vi "GUI.vi"(9 "GUI Builder in":refnum<class "GUI Builder.lvclass">) -> ()   [LabVIEW 2021, in "App-Builder Library.lvlib" / "GUI Builder.lvclass"]
uses:
  GUI Builder.lvclass
  Builder/App descriptions.ctl
  Builder/Build Type.ctl
  GUI Builder.lvclass/GUI Builder.ctl
  Builder/Builder.lvclass
panel:
  in  "Application found":T1[](array[typedef])
  out "update":bool
  in  "Build button":bool
  # "Build Name"
  # "Type"
  # "Current Version"
  # "Next Version"
  # "Build?"
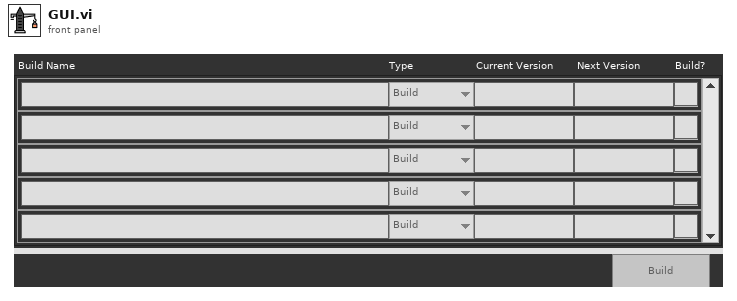
[diagram p1: front panel]
types:
  T1 = typedef "App-Builder Library.lvlib/Builder.lvclass/App descriptions.ctl" = cluster{"App Name":string, "Build Type":T2, "Current Version":string, "Next Version":string, "Check":bool}
  T2 = typedef "App-Builder Library.lvlib/Builder.lvclass/Build Type.ctl" = enum16{"Major", "Minor", "Fix", "Build"}
  T3 = enum8{"Enabled", "Disabled", "Disabled and Grayed Out"}
  T4 = typedef "NI_App_Builder_API.lvlib/Build Specification Version.ctl" = cluster{"Major":u16, "Minor":u16, "Fix":u16, "Build":u16}
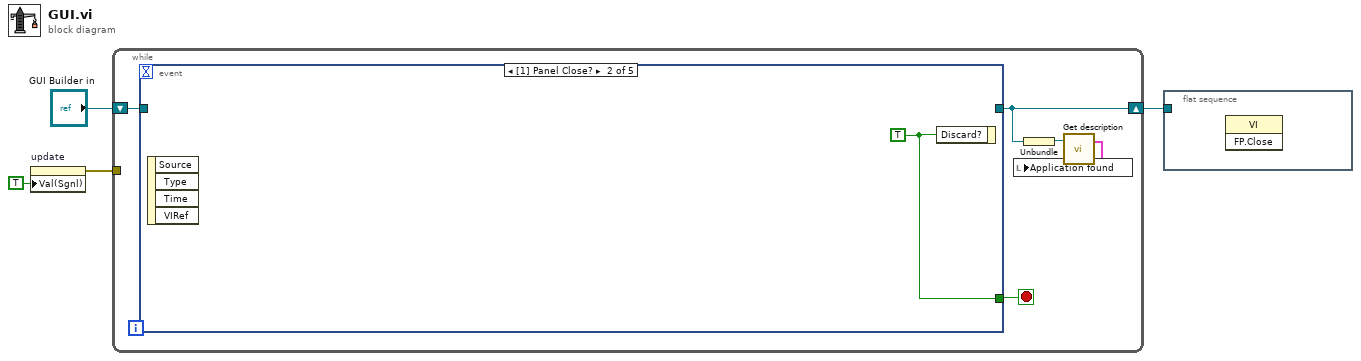
[diagram p0: block diagram]
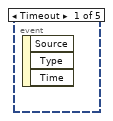
[diagram p2: hidden frame]
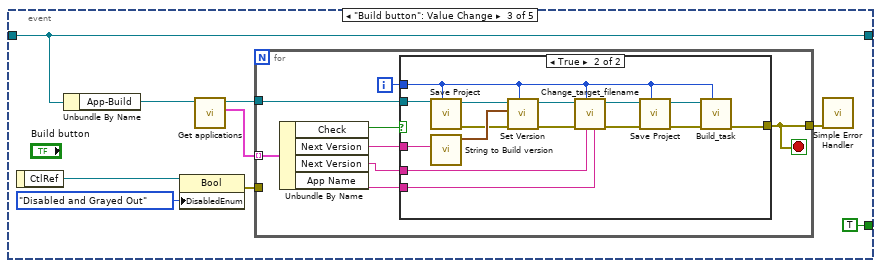
[diagram p3: hidden frame]
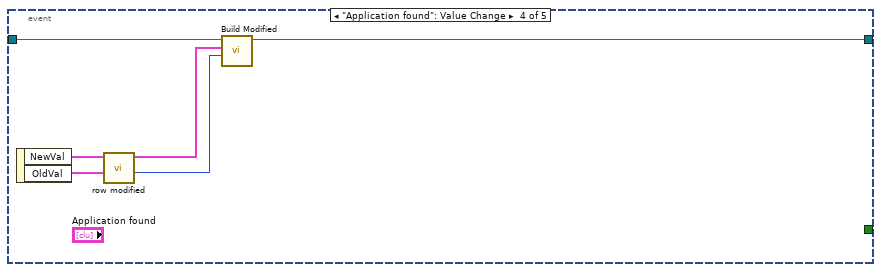
[diagram p5: hidden frame]
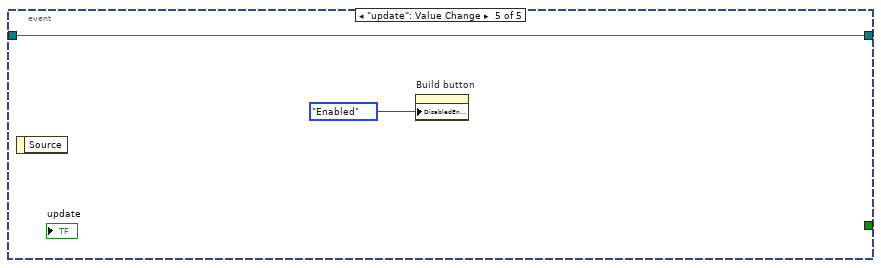
[diagram p6: hidden frame]
diagram:
  n1 = property on="update" class="Bool (strict)"("Val(Sgnl)"=TRUE ("Value (Signaling)")) -> (error out=w2:errorcluster)  [unwired: 2 in, 1 out]
  n2 = while {
    shift-right: [w6] -> w1
    shift-left: "GUI Builder in" -> [w8]
    tunnel: w2 -> [_]
    stop <- w9 stop-if-true
    n3 = event shown="[1] Panel Close?" {
      selector: _ -> [_ _ _ _ _]
      dyn-events: _ -> [_ _ _ _ _]
      timeout: _ -> [_ _ _ _ _]
      tunnel: [_ w10 TRUE ("Discard?") _ _] -> w9
      tunnel: w8 -> [_ _ w19 w46 w50]
      tunnel: [_ _ w19 w44 w50] -> w6
      event Timeout {
        n4 = event-data() -> ()  [unwired: 1 in, 3 out]
      }
      event Panel Close? {
        w10 = TRUE ("Discard?")
        n5 = event-data() -> ()  [unwired: 1 in, 4 out]
        n6 = event-data("Discard?"=w10) -> ()  [unwired: 1 in, 1 out]
      }
      event "Build button": Value Change {
        n7 = event-data() -> ("CtlRef"=w15:refnum<vi>)  [unwired: 1 in]
        n8 = Unbundle By Name(w19) -> ("App-Build"=w18:refnum<class "Builder.lvclass">)
        n9 = property class="Bool"(reference=w15, "DisabledEnum"=T3."Disabled and Grayed Out" ("Disabled")) -> (error out=w13:errorcluster)  [unwired: 1 in, 1 out]
        n10 = call "Get applications.vi"("Builder in"=w18) -> ("Applications"=w16:T1[], "Builder out"=w17:refnum<class "Builder.lvclass">)  [unwired: 9 in]
        n11 = for {
          tunnel: [w22] -> w11
          tunnel: w17 -> [w27]
          tunnel: w16 -> [w26] mode=indexing
          tunnel: w13 -> [_]
          i -> [w24]
          stop <- w22 stop-if-true
          n12 = Unbundle By Name(w26) -> ("Check"=w25:bool, "Next Version"=w23:string, "Next Version"=w20:string, "App Name"=w21:string)
          n13 = case shown="True" w25 {
            tunnel: [_ w32] -> w22
            tunnel: w27 -> [_ w38]
            tunnel: w24 -> [_ w30]
            tunnel: w23 -> [_ w40]
            tunnel: w21 -> [_ w29]
            tunnel: w20 -> [_ w28]
            frame False {
            }
            frame True {
              n14 = call "Save Project.vi"("index"=w30, "Builder in"=w38) -> ("error out"=w31:errorcluster, "Builder out"=w37:refnum<class "Builder.lvclass">)  [unwired: 8 in]
              n15 = call "String to Build version.vi"("Build Version (String)"=w40) -> ("Build Version"=w39:T4)  [unwired: 10 in]
              n16 = call "Set Version.vi"("Index"=w30, "error in"=w31, "Build Version"=w39, "Builder in"=w37) -> ("error out"=w41:errorcluster, "Builder out"=w42:refnum<class "Builder.lvclass">)  [unwired: 6 in]
              n17 = call "Change_target_filename.vi"("App Name"=w29, "New Version"=w28, "index"=w30, "error in (no error)"=w41, "Builder in"=w42) -> ("error out"=w36:errorcluster, "Builder out"=w35:refnum<class "Builder.lvclass">)  [unwired: 5 in]
              n18 = call "Save Project.vi"("index"=w30, "error in"=w36, "Builder in"=w35) -> ("error out"=w33:errorcluster, "Builder out"=w34:refnum<class "Builder.lvclass">)  [unwired: 7 in]
              n19 = call "Build_task.vi"("index"=w30, "error in"=w33, "Builder in"=w34) -> ("error out"=w32:errorcluster)  [unwired: 6 in, 2 out]
            }
          }
        }
        n20 = call <vilib>:"Simple Error Handler.vi"("error in (no error)"=w11) -> ()  [unwired: 4 in, 5 out]
      }
      event "Application found": Value Change {
        n21 = event-data() -> ("NewVal"=w48:T1[], "OldVal"=w47:T1[])  [unwired: 1 in]
        n22 = call "row modified.vi"("OldVal"=w47, "NewVal"=w48) -> ("Index"=w43:i32, "Value Modified"=w45:T1)  [unwired: 8 in]
        n23 = call "Build Modified.vi"("index"=w43, "build modified"=w45, "GUI Builder in"=w46) -> ("GUI Builder out"=w44:refnum<class "GUI Builder.lvclass">)  [unwired: 8 in]
      }
      event "update": Value Change {
        n24 = event-data() -> ()  [unwired: 1 in, 1 out]
        n25 = property on="Build button" class="Bool"("DisabledEnum"=T3."Enabled" ("Disabled")) -> ()  [unwired: 2 in, 2 out]
      }
    }
    n26 = Unbundle(w6) -> (w5:refnum<class "Builder.lvclass">)
    n27 = call "Get description.vi"("Builder in"=w5) -> ("Applications"=w7:T1[])  [unwired: 2 in]
    n28 = local write "Application found"(w7) -> ()
  }
  n29 = flat-sequence {
    tunnel: w1 -> [_]
    frame #0 {
      n30 = invoke class="VI" method="FP.Close"() -> ()  [unwired: 3 in, 3 out]
    }
  }
